vi "kvCanReadStatus.vi"(0 "Channel Handle (input only)":i32, 1 "error in (no error)":errorcluster) -> (2 "Channel Handle (ouput only)":i32, 3 "Status Flags":u32 format="%.0x", 4 "error out":errorcluster)   [LabVIEW 2022 SP3]
doc: "Returns the status for the specified circuit. flags points to a longword which receives a combination of the canSTAT_xxx flags.\n\nNote: canReadStatus returns the latest known status of the specified circuit. If a status change happens precisely when canReadStatus is called, it may not be reflected in the returned result."
uses:
  canlib32.dll
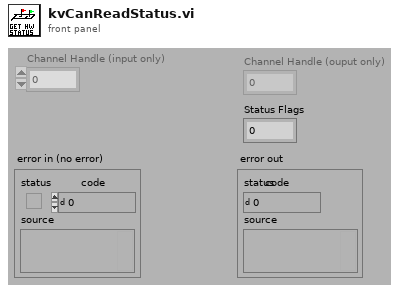
[diagram p1: front panel]
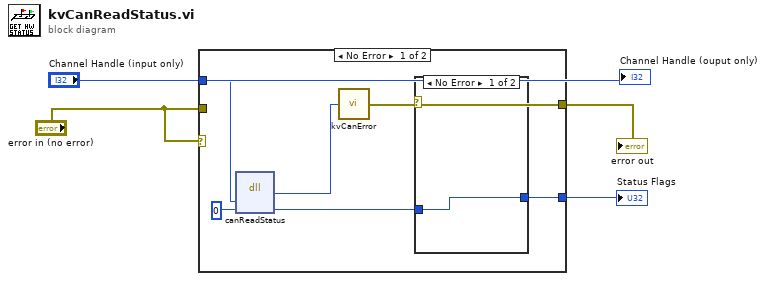
[diagram p0: block diagram]
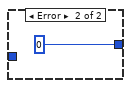
[diagram p2: hidden frame]
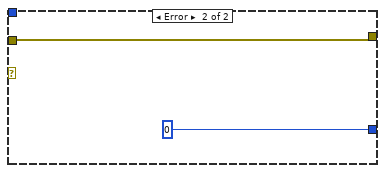
[diagram p3: hidden frame]
diagram:
  n1 = case shown="No Error" "error in (no error)" {
    tunnel: "error in (no error)" -> [_ w14]
    tunnel: "Channel Handle (input only)" -> [w9 _]
    tunnel: [w7 w14] -> w2
    tunnel: [w6 0] -> w1
    frame No Error {
      n2 = dll-call lib="canlib32.dll" fn="canReadStatus" label="Call CanReadStatus"("channelHandle"=w9, "flags"=0) -> (w10:i32, "flags"=w5:u32)  [unwired: 4 in, 2 out]
      n3 = call "kvCanError.vi"("error code"=w10) -> ("error out"=w7:errorcluster)
      n4 = case shown="No Error" w7 {
        tunnel: [w11 0] -> w6
        tunnel: w5 -> [w11 _]
        frame No Error {
        }
        frame Error {
        }
      }
    }
    frame Error {
    }
  }
  "error out" <- w2
  "Status Flags" <- w1
  "Channel Handle (ouput only)" <- "Channel Handle (input only)"
